vi "XYZ to 2D Array.vi"(7 "IntensityGraph in":refnum<vi>, 8 "2D Array Settings":T1={"x Max"=270.0, "x Min"=65.0, "x step size"=2.5, "y Max"=320.0, "y Min"=5.0, "y step size"=2.5} {"y step size" format="%#_13g"; "y Min" format="%#_13g"; "y Max" format="%#_13g"; "x step size" format="%#_13g"; "x Min" format="%#_13g"; "x Max" format="%#_13g"}, 9 "Z":dbl[](array[numeric]), 10 "Y":dbl[](array[numeric]), 11 "X":dbl[](array[numeric])) -> (1 "Y Array":dbl[](array[numeric]), 2 "X Array":dbl[](array[numeric]), 3 "2D Array out":dbl[][](array[numeric]))   [LabVIEW 2016]
uses:
  <userlib>/LevyLab/Graph Utilities/graph_utilities.lvclass
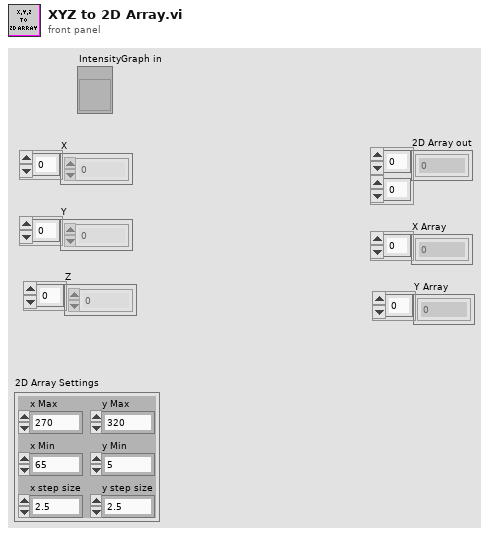
[diagram p1: front panel]
types:
  T1 = cluster{"x Max":dbl, "x Min":dbl, "x step size":dbl, "y Max":dbl, "y Min":dbl, "y step size":dbl}
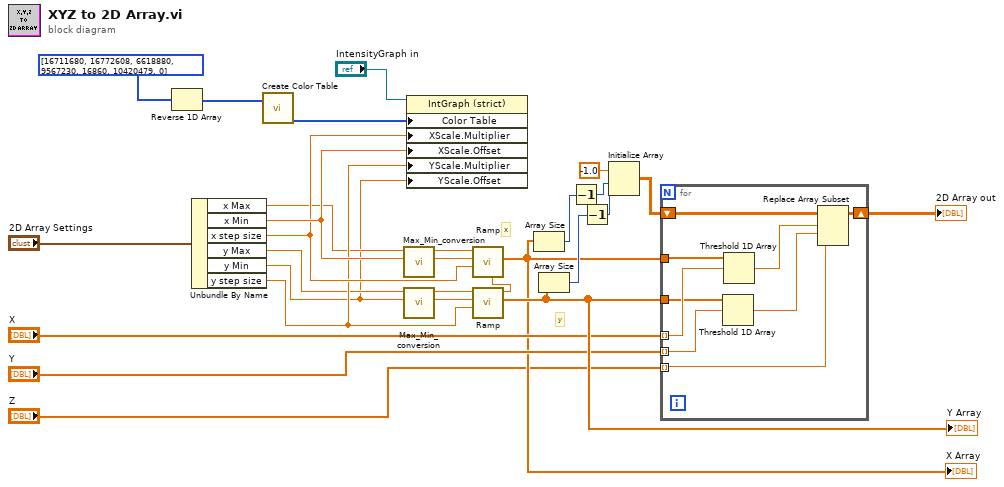
[diagram p0: block diagram]
diagram:
  # "x"
  # "y"
  n1 = Reverse 1D Array(array=u32[] [16711680, 16772608, 6618880, 9567230, 16860, 10420479, 0] ("color scale")) -> (reversed array=w13:u32[])
  n2 = Unbundle By Name("2D Array Settings") -> ("x Max"=w24:dbl, "x Min"=w28:dbl, "x step size"=w27:dbl, "y Max"=w25:dbl, "y Min"=w1:dbl, "y step size"=w26:dbl)
  n3 = call <userlib>:"Create Color Table.vi"("Colors []"=w13) -> ("Color Tbl"=w2:u32[])  [unwired: 1 in, 3 out]
  n4 = call <userlib>:"Max_Min_conversion.vi"("Min"=w28, "Max"=w24) -> ("offset"=w9:dbl, "Amplitude"=w8:dbl)  [unwired: 8 in]
  n5 = call <userlib>:"Max_Min_conversion.vi"("Min"=w1, "Max"=w25) -> ("offset"=w10:dbl, "Amplitude"=w11:dbl)  [unwired: 8 in]
  n6 = property on="Property Node" class="IntGraph (strict)"(reference="IntensityGraph in", "Color Table"=w2, "XScale.Multiplier"=w27, "XScale.Offset"=w28, "YScale.Multiplier"=w26, "YScale.Offset"=w1) -> ()  [unwired: 1 in, 2 out]
  n7 = call <userlib>:"Ramp.vi"("step size"=w26, "offset"=w10, "amplitude"=w11) -> ("Waveform Graph"=w19:dbl[], "element"=w12:dbl)  [unwired: 6 in, 1 out]
  "Y Array" <- w19
  n8 = call <userlib>:"Ramp.vi"("i"=w12, "step size"=w27, "offset"=w9, "amplitude"=w8) -> ("Waveform Graph"=w5:dbl[])  [unwired: 5 in, 2 out]
  "X Array" <- w5
  n9 = Array Size(array=w5) -> (size(s)=w21:i32)
  n10 = Array Size(array=w19) -> (size(s)=w22:i32)
  n11 = Decrement(x=w21) -> (x-1=w17:i32)
  n12 = Decrement(x=w22) -> (x-1=w18:i32)
  n13 = Initialize Array(-1.0 ("element"), w17, w18) -> (w20:dbl[][])
  n14 = for {
    tunnel: "X" -> [w36] mode=indexing
    tunnel: "Y" -> [w34] mode=indexing
    tunnel: "Z" -> [w33] mode=indexing
    tunnel: w5 -> [w37]
    tunnel: w19 -> [w35]
    shift-right: [w30] -> w16
    shift-left: w20 -> [w29]
    n15 = Threshold 1D Array(2:w34, 3:w35) -> (0:w32:dbl)  [unwired: 1 in]
    n16 = Threshold 1D Array(2:w36, 3:w37) -> (0:w31:dbl)  [unwired: 1 in]
    n17 = Replace Array Subset(array=w29, new element=w33, index (row)=w31, index (col)=w32) -> (w30:dbl[][])
  }
  "2D Array out" <- w16
